vi "PTSequencer.set stop conditions.vi"(0 "i ref in":refnum<vi>, 1 "stop conditions":T1[](array[typedef]), 3 "ms timeout (10000)":i32=10000, 4 "use stop conditions":bool, 5 "error in (no error)":errorcluster) -> (14 "i ref out":refnum<vi>, 17 "timed out":bool, 19 "error out":errorcluster)   [LabVIEW 2014, in "PTSequencer.lvlib"]
uses:
  PTSequencer.lvlib
  PTSequencer.DIM service condition.ctl
  CSCore/CSSystem/CoreDefs/CoreDefs.rawDataType.ctl
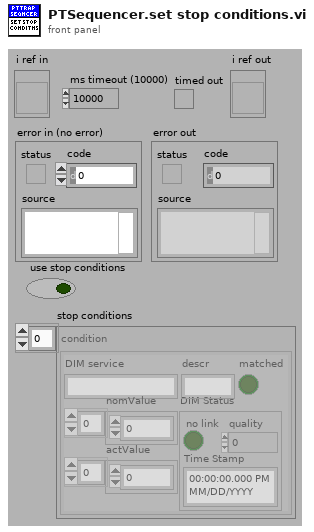
[diagram p1: front panel]
types:
  T1 = typedef "PTSequencer.lvlib/PTSequencer.DIM service condition.ctl" = cluster{"DIM service":string, "descr":string, "nomValue":T2, "actValue":T2, "matched":bool, "DIM Status":cluster{"no link":bool, "quality":i32, "Time Stamp":timestamp}}
  T2 = typedef "CoreDefs.rawDataType.ctl" = i8[]
  T3 = typedef "PTSequencer.lvlib/PTSequencer.i attribute.ctl" = cluster{"subsequence":bool, "mode":T4, "i step":i32, "nofLoops":i32, "i loop":i32, "Running":bool, "Paused":bool, "step done":bool, "loop done":bool, "seq done":bool, "DIM IDs":cluster{"step done":i32, "loop done":i32, "seq done":i32, "i step":i32, "i loop":i32}, "use stop conditions":bool, "stop conditions":T1[], "Step List":T5[], "DIM subsriptions":string[], "stop cond indexes":i32[], "step cond indexes":cluster{"step condition IDs":cluster{"step ID":i32, "condition ID":i32}[]}[], "Delay Start Time":timestamp, "status":string, "stopping":bool}
  T4 = typedef "PTSequencer.lvlib/PTSequencer.mode.ctl" = enum16{"single", "loop", "for loop"}
  T5 = typedef "PTSequencer.lvlib/PTSequencer.step.ctl" = cluster{"description":string, "object parameters":cluster{"object":string, "selector":string, "descriptor":string, "data":T2, "subsequence":bool, "call mode":enum16{"Simple DIM", "Synchronous"}, "data in":T2}, "result action":cluster{"check":bool, "passed":enum16{"Next", "Previous", "Repeat", "Jump"}, "failed":enum16{"Next", "Previous", "Repeat", "Jump"}, "jumpID_passed":i32, "jumpID_failed":i32}, "conditions":T1[], "fulfilled ":bool, "use delay":bool, "delay time (s)":dbl, "ID":i32}
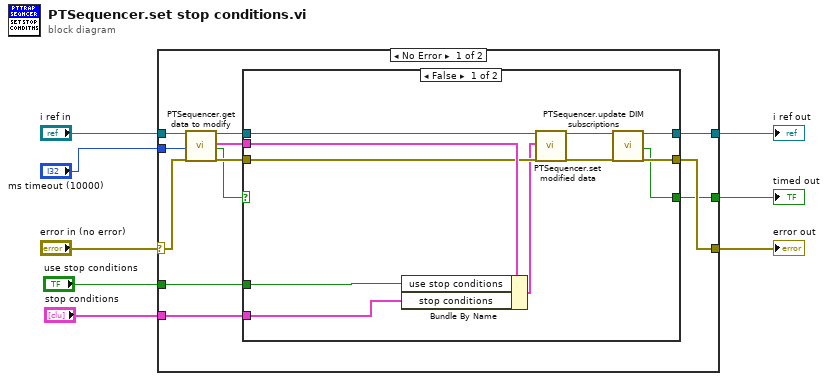
[diagram p0: block diagram]
diagram:
  n1 = case shown="No Error" "error in (no error)" {
    selector: "error in (no error)" -> [w15 w35]
    tunnel: "i ref in" -> [w20 w36]
    tunnel: [w13 w36] -> w6
    tunnel: [w12 w35] -> w5
    tunnel: "ms timeout (10000)" -> [w14 _]
    tunnel: [w11 _] -> w3
    tunnel: "use stop conditions" -> [w10 _]
    tunnel: "stop conditions" -> [w9 _]
    frame No Error {
      n2 = call "PTSequencer.get data to modify.vi"("i ref in"=w20, "ms timeout (10000)"=w14, "error in (no error)"=w15) -> ("i ref out"=w19:refnum<vi>, "i attribute"=w17:T3, "timed out"=w16:bool, "error out"=w18:errorcluster)  [unwired: 13 in]
      n3 = case shown="False" w16 {
        selector: w16 -> [_ w32]
        tunnel: w19 -> [w30 w34]
        tunnel: w18 -> [w29 w33]
        tunnel: w17 -> [w31 _]
        tunnel: [w24 w34] -> w13
        tunnel: [w25 w33] -> w12
        tunnel: [w23 w32] -> w11
        tunnel: w10 -> [w22 _]
        tunnel: w9 -> [w21 _]
        frame False {
          n4 = Bundle By Name(cluster=w31, "use stop conditions"=w22, "stop conditions"=w21) -> (w28:T3)
          n5 = call "PTSequencer.set modified data.vi"("i ref in"=w30, "CLASS.i attribute"=w28, "error in (no error)"=w29) -> ("i ref out"=w26:refnum<vi>, "error out"=w27:errorcluster)  [unwired: 15 in]
          n6 = call "PTSequencer.update DIM subscriptions.vi"("i ref in"=w26, "error in"=w27) -> ("i ref out"=w24:refnum<vi>, "timed out"=w23:bool, "error out"=w25:errorcluster)  [unwired: 15 in]
        }
        frame True {
        }
      }
    }
    frame Error {
    }
  }
  "error out" <- w5
  "i ref out" <- w6
  "timed out" <- w3
